vi "Set Network Adapter Settings.vi"(8 "error in (no error)":errorcluster, 10 "Network Adapter Settings":T1[](array[typedef]) {"IP Address Request Mode" items=["Static"=1, "DHCP/Link Local"=2, "Link-Local Only"=4, "DHCP Only"=8]; "Adapter Type" items=["Disabled"=1, "TCP/IP Ethernet"=2, "Deterministic"=4, "EtherCAT"=8, "TCP/IP WLAN Connect"=32, "TCP/IP WLAN Create"=64]; "Adapter Mode" items=["Disabled"=1, "TCP/IP Ethernet"=2, "Deterministic"=4, "EtherCAT"=8, "TCP/IP WLAN Connect"=32, "TCP/IP WLAN Create"=64]}, 11 "Device in":refnum<class "Device.lvclass">=refnum) -> (0 "error out":errorcluster, 3 "Device out":refnum<class "Device.lvclass">)   [LabVIEW 2016]
uses:
  Device.lvclass
  Controls/NetworkAdapterSettings.ctl
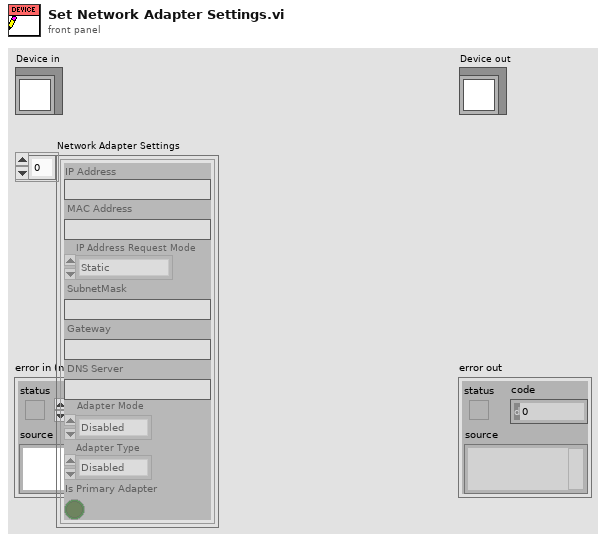
[diagram p1: front panel]
types:
  T1 = typedef "RT Management.lvlib/Device.lvclass/NetworkAdapterSettings.ctl" = cluster{"IP Address":string, "MAC Address":string, "IP Address Request Mode":u32, "SubnetMask":string, "Gateway":string, "DNS Server":string, "Adapter Mode":u32, "Adapter Type":u32, "Is Primary Adapter":bool}
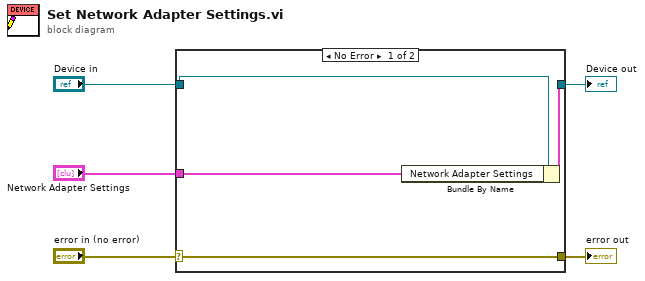
[diagram p0: block diagram]
diagram:
  n1 = case shown="No Error" "error in (no error)" {
    selector: "error in (no error)" -> [w9 w10]
    tunnel: [w9 w10] -> w4
    tunnel: [w7 w11] -> w2
    tunnel: "Device in" -> [w8 w11]
    tunnel: "Network Adapter Settings" -> [w6 _]
    frame No Error {
      n2 = Bundle By Name(cluster=w8, "Network Adapter Settings"=w6) -> (w7:cluster{})
    }
    frame Error {
    }
  }
  "error out" <- w4
  "Device out" <- w2
